vi "SonarBrake - Rev2.vi"() -> ()   [LabVIEW 2018]
uses:
  <vilib>/Platform/TimedLoop/XDataNode/timing_clust.ctl
  <vilib>/Platform/TimedLoop/XDataNode/nitl_modes.ctl
  <vilib>/Platform/TimedLoop/XDataNode/wakeup.ctl
  <vilib>/addons/control/pid/pid.llb/PID (DBL).vi
  <vilib>/platform/TimedLoop/XDataNode/XDataNode.xnode
  <vilib>/Platform/TimedLoop/XDataNode/XDNodeRunTimeDep.lvlib
  <vilib>/addons/control/pid/NI_PID_pid.lvlib
panel:
  in  "Reset":bool
  out "Diag":cluster{i32, i16, dbl, i16}(graph)={3, 0, 0.43266588939999995, 1}
  in  "Read Enable":T1={"Cal Status"=TRUE, "Orientation"=TRUE, "Gyro"=FALSE, "Accelerometer"=FALSE, "Quanterion"=FALSE, "Accel Mode"=enum."Linear", "Magnetometer"=FALSE, "Register Mode"=enum."Quaternion"}
  in  "Tab Control":enum32{"Sonar"}(tab)
  in  "Tol (sec)":dbl=0.25 format="%#_13g"
  in  "Tol (in)":dbl=1.1
  out "Arrived":bool
  out "Sonar Error":dbl=-4.3266588939999995
  in  "Rate Thresh":dbl=100.0 format="%#_13g"
  out "OOR":bool
  out "Mode":bool=TRUE
  in  "hi limit":dbl=200.0
  out "Strobe":bool
  in  "standoff":dbl=5.0 format="%.2f"
  out "Sonar Left":cluster{"Filtered":dbl, dbl}(graph)={"Filtered"=12.326658894, 12.326658894}
  out "Sonar Late?":bool
  out "Period":i64=40
  in  "Reset Enc":bool
  out "Enc":dbl=-31.431918913398693
  in  "Hyster":dbl=0.1 format="%#_13g"
  out "State":i32=3
  in  "reset IMU":bool
  in  "Test?":bool
  in  "clamp":cluster{"output high":dbl, "output low":dbl}={"output high"=1.0, "output low"=-1.0} {"output low" format="%.2f"; "output high" format="%.2f"}
  in  "Trans":dbl=14.0
  out "close":bool=TRUE
  in  "PID Sonar":T2={"proportional gain (Kc)"=0.035, "integral time (Ti, min)"=0.0, "derivative time (Td, min)"=0.001} {"derivative time (Td, min)" format="%.5f"; "integral time (Ti, min)" format="%.3f"; "proportional gain (Kc)" format="%.3f"}
  in  "Use Enc?":bool
  out "Sonar PID":cluster{"setpoint":dbl, "Filtered":dbl, i16}(graph)={"setpoint"=8.0, "Filtered"=12.326658894, 0}
  out "PID error":dbl=4.3266588939999995
  in  "scale enc":dbl=-0.04
  in  "db":dbl=0.04
  # "Real Time Data Repair"
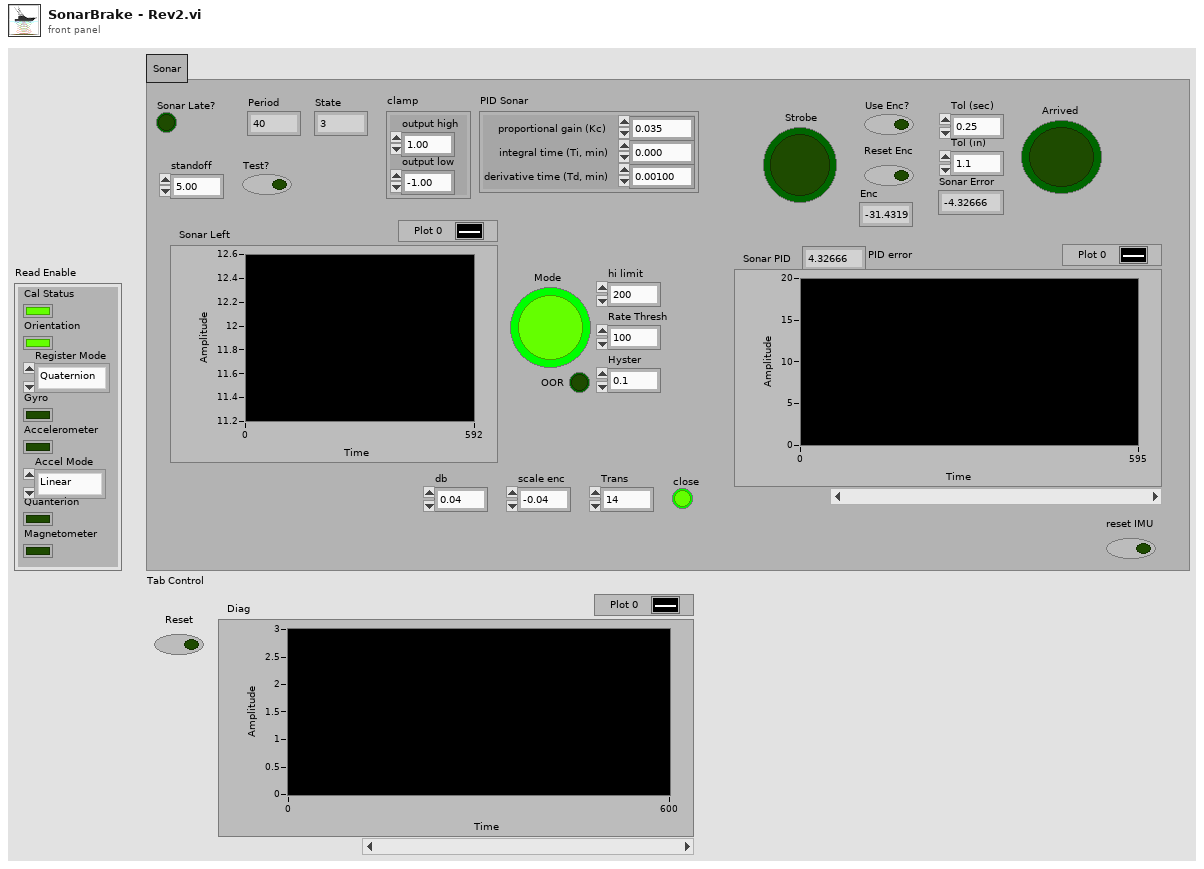
[diagram p1: front panel]
types:
  T1 = cluster{"Cal Status":bool, "Orientation":bool, "Gyro":bool, "Accelerometer":bool, "Quanterion":bool, "Accel Mode":enum8{"Raw Data", "Linear", "Gravity"}, "Magnetometer":bool, "Register Mode":enum8{"Euler", "Quaternion"}}
  T2 = cluster{"proportional gain (Kc)":dbl, "integral time (Ti, min)":dbl, "derivative time (Td, min)":dbl}
  T3 = typedef "ImuDevRef.ctl" = cluster{"I2CDevRef":T4, "Valid Cal File?":bool}
  T4 = typedef "WPI_I2CDevRef.ctl" = cluster{"DevStatus":errorcluster, "Device Address":u8, "Handle":i32, "I2C Bus":T5}
  T5 = typedef "i2c_bus.ctl" = enum16{"I2C On-Board", "I2C MXP", "Invalid"}
  T6 = typedef "XDNodeRunTimeDep.lvlib/timing_clust.ctl" = cluster{"Expected End [f-1]":u64, "Actual End [f-1]":u64, "Finished Late? [f-1]":bool, "Expected End [i-1]":u64, "Actual End [i-1]":u64, "Finished Late? [i-1]":bool, "Expected Start [i]":u64, "Actual Start [i]":u64, "Expected Start [f]":u64, "Actual Start [f]":u64, "Source Name":string, "Structure Name":string, "Period":i64, "Deadline":i64, "Offset":i64, "Start":i64, "Priority":i32, "Timeout":i32, "Mode":T7, "Wakeup Reason":T8, "Error":errorcluster, "Source Type":string, "Secondary Source Type":string, "Global End Time":u64, "Global Start Time":u64, "Frame Duration":u64, "Iteration Duration":u64, "Assigned CPU":i32, "I/O Scan Engine Mode":u32}
  T7 = typedef "XDNodeRunTimeDep.lvlib/nitl_modes.ctl" = enum32{"No Change", "Process missed periods, maintain original phase", "Discard missed periods, maintain original phase", "Process missed periods, ignore original phase", "Discard missed periods, ignore original phase"}
  T8 = typedef "XDNodeRunTimeDep.lvlib/wakeup.ctl" = enum32{"Normal", "Aborted", "Asynchronous wakeup", "Timing source error", "Timed loop error", "Timeout"}
  T9 = typedef "WPI_AnalogChannelDevRef.ctl" = cluster{"DevStatus":errorcluster, "Analog Channel":T10}
  T10 = typedef "FPGA_AIChannel.ctl" = enum8{"AI 0", "AI 1", "AI 2", "AI 3", "AI MXP 0", "AI MXP 1", "AI MXP 2", "AI MXP 3", "Invalid"}
  T11 = cluster{"Yaw":dbl, "Roll":dbl, "Pitch":dbl, "Yaw Wind":dbl, "Roll Wind":dbl, "Pitch Wind":dbl}
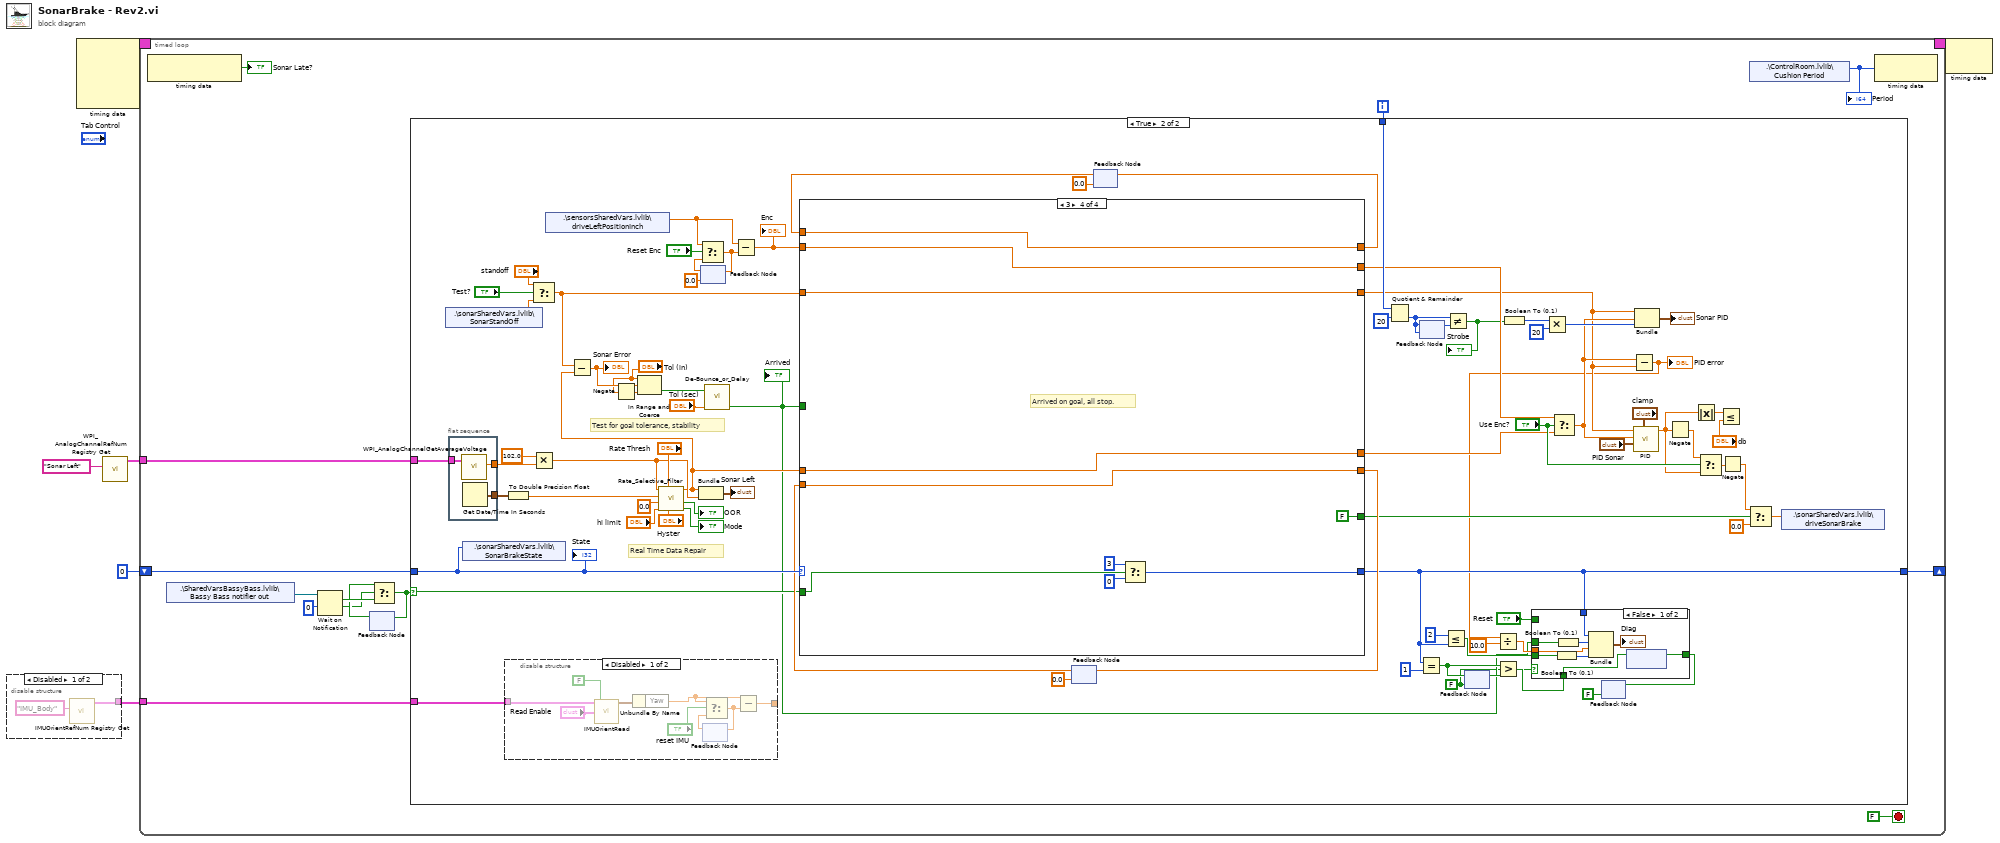
[diagram p0: block diagram]
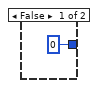
[diagram p3: hidden frame]
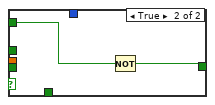
[diagram p4: hidden frame]
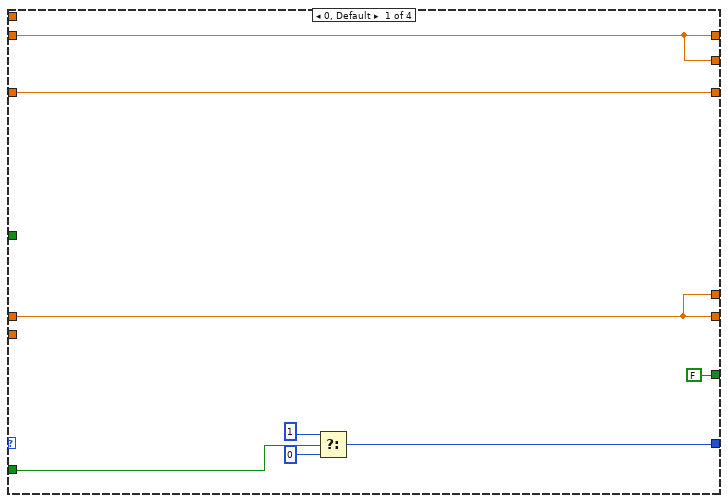
[diagram p6: hidden frame]
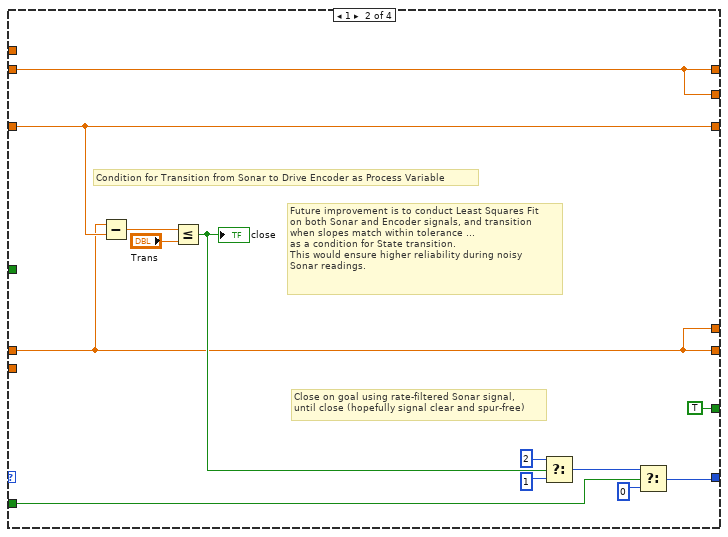
[diagram p7: hidden frame]
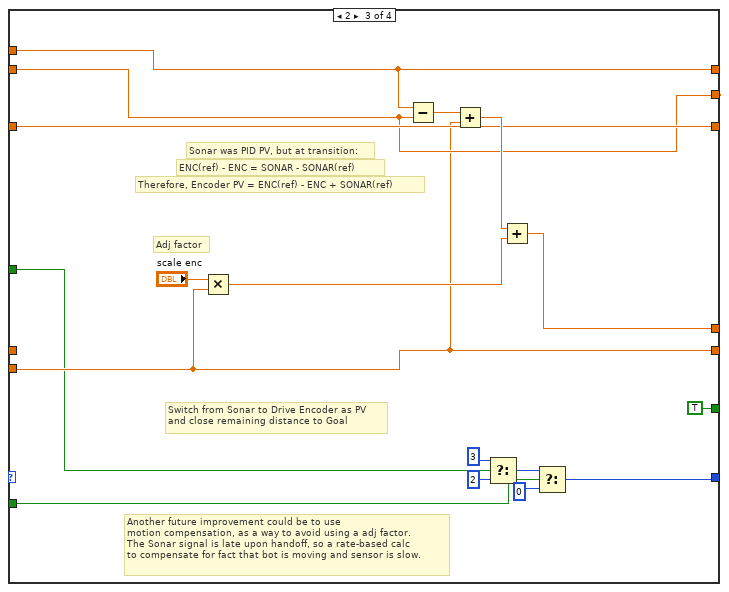
[diagram p8: hidden frame]
diagram:
  n1 = disable-structure shown="Disabled" {
    disable-tunnel: [w7 _] -> w1
    frame Disabled {
      n2 = call <userlib>:"IMUOrientRefNum Registry Get.vi"("refnum name"="IMU_Body") -> ("IMUDevRef out"=w7:T3)  [unwired: 9 in, 1 out]
    }
    frame Enabled {
    }
  }
  n3 = node-c288() -> (w6:T6)  [unwired: 4 in]
  n4 = call <vilib>:"WPI_AnalogChannelRefNum Registry Get.vi"("refnum name"="Sonar Left") -> ("AIDeviceRef"=w3:T9)  [unwired: 9 in, 1 out]
  n5 = timed-loop {
    timing: w6 -> [_]
    timing-out: [_] -> w5
    tunnel: w3 -> [w21]
    shift-right: [w15] -> _
    shift-left: 0 -> [w16]
    tunnel: w1 -> [w17]
    i -> [w19]
    stop <- FALSE stop-if-true
    n6 = node-c288() -> (→"Sonar Late?":bool)  [unwired: 1 in]
    n7 = shared-variable ".\\SharedVarsBassyBass.lvlib\\Bassy Bass notifier out"() -> (w14:refnum<notifier>)  [unwired: 1 in, 1 out]
    n8 = Wait on Notification(notifier=w14, timeout in ms (-1)=0) -> (notification=w12:bool, timed out?=w10:bool)  [unwired: 2 in, 2 out]
    n9 = feedback #1() -> (w11:bool)  [unwired: 1 in]
    n10 = Select(t=w11, s=w10, f=w12) -> (s? t:f=w9:bool)
    n11 = feedback-in #1(w9) -> ()
    n12 = case shown="True" w9 {
      selector: w9 -> [_ w30]
      tunnel: w21 -> [_ w101]
      tunnel: w19 -> [_ w97]
      tunnel: w17 -> [_ w74]
      tunnel: w16 -> [_ w68]
      tunnel: [0 ("t") w36] -> w15
      frame False {
      }
      frame True {
        w24 = FALSE ("Shock")
        # "Real Time Data Repair"
        # "Test for goal tolerance, stability"
        n13 = shared-variable ".\\sonarSharedVars.lvlib\\SonarStandOff"() -> (w71:dbl)  [unwired: 1 in, 1 out]
        n14 = flat-sequence {
          tunnel: [w124] -> w87
          tunnel: w101 -> [w123]
          tunnel: [w122] -> w94
          frame #0 {
            n15 = call <vilib>:"WPI_AnalogChannelGetAverageVoltage.vi"("AIDeviceRef"=w123) -> ("Voltage"=w124:dbl)  [unwired: 8 in, 2 out]
            n16 = Get Date/Time In Seconds() -> (seconds since 1Jan1904=w122:timestamp)
          }
        }
        n17 = shared-variable ".\\sonarSharedVars.lvlib\\SonarBrakeState"(w68) -> ()  [unwired: 1 in, 1 out]
        n18 = disable-structure shown="Disabled" {
          disable-tunnel: w74 -> [w114 _]
          disable-tunnel: [w113 _] -> _
          frame Disabled {
            n19 = call <userlib>:"IMUOrientRead.vi"("IMU Dev Ref"=w114, "Orient Reset (Wind)"=FALSE, "Read Enable"="Read Enable") -> ("Orient Y/R/P"=w119:T11)  [unwired: 5 in, 7 out]
            n20 = Unbundle By Name(w119) -> ("Yaw"=w115:dbl)
            n21 = feedback #2() -> (w118:dbl)  [unwired: 1 in]
            n22 = Select(t=w115, s="reset IMU", f=w118) -> (s? t:f=w117:dbl)
            n23 = feedback-in #2(w117) -> ()
            n24 = Subtract(x=w115, y=w117) -> (x-y=w113:dbl)
          }
          frame Enabled {
          }
        }
        n25 = To Double Precision Float(number=w94) -> (double precision float=w93:dbl)
        n26 = Select(t="standoff", s="Test?", f=w71) -> (s? t:f=w72:dbl)
        n27 = Multiply(x=102.0, y=w87) -> (x*y=w82:dbl)
        n28 = shared-variable ".\\sensorsSharedVars.lvlib\\driveLeftPositionInch"() -> (w75:dbl)  [unwired: 1 in, 1 out]
        n29 = Negate(x="Tol (in)") -> (-x=w85:dbl)
        n30 = call <userlib>:"Rate_Selective_Filter.vi"("Hyster"="Hyster", "Rate Thresh"="Rate Thresh", "hi limit"="hi limit", "lo limit"=0.0, "Time"=w93, "Distance"=w82) -> ("Mode"=→"Mode":bool, "OOR"=→"OOR":bool, "Filtered"=w76:dbl)  [unwired: 1 in]
        n31 = Subtract(x=w72, y=w76) -> (x-y=w86:dbl)
        "Sonar Error" <- w86
        n32 = In Range and Coerce(upper limit="Tol (in)", x=w86, lower limit=w85) -> (In Range?=w25:bool)  [unwired: 1 out]
        n33 = Bundle("Filtered"=w76, w82) -> (→"Sonar Left":cluster{"Filtered":dbl, dbl})  [unwired: 1 in]
        n34 = feedback #3(0.0) -> (w79:dbl)
        n35 = Select(t=w75, s="Reset Enc", f=w79) -> (s? t:f=w77:dbl)
        n36 = feedback-in #3(w77) -> ()
        n37 = call <userlib>:"De-Bounce_or_Delay.vi"("Eval Period (sec)"="Tol (sec)", "Signal Input"=w25) -> ("Stable"=w26:bool)  [unwired: 9 in]
        "Arrived" <- w26
        n38 = Subtract(x=w75, y=w77) -> (x-y=w78:dbl)
        "Enc" <- w78
        n39 = feedback #4(0.0 ("Filtered")) -> (w54:dbl)
        n40 = feedback #5(0.0) -> (w57:dbl)
        n41 = case shown="3" w68 {
          tunnel: [w131 w145 w161 w164] -> w36
          tunnel: w30 -> [w129 w144 w160 w163]
          tunnel: w72 -> [w128 w137 w151 w169]
          tunnel: w78 -> [w126 w134 w150 w170]
          tunnel: w76 -> [w125 w133 _ w168]
          tunnel: w26 -> [_ _ w147 _]
          tunnel: [w126 w134 w152 w171] -> w59
          tunnel: [w128 w137 w151 w169] -> w34
          tunnel: [w125 w133 w148 w167] -> w56
          tunnel: [w125 w133 w149 w168] -> w52
          tunnel: [w126 w134 w150 w170] -> w53
          tunnel: w57 -> [_ _ w152 w171]
          tunnel: w54 -> [_ _ w148 w167]
          tunnel: [FALSE TRUE TRUE FALSE] -> w48
          frame 0, Default {
            n42 = Select(t=1, s=w129, f=0) -> (s? t:f=w131:i32)
          }
          frame 1 {
            # "Close on goal using rate-filtered Sonar signal,\nuntil close (hopefully signal clear and spur-free)"
            # "Future improvement is to conduct Least Squares Fit\non both Sonar and Encoder signals, and transition\nwhen slopes match within tolerance ...\nas a condition for State transition.\nThis would ensure higher reliability during noisy\nSonar readings."
            # "Condition for Transition from Sonar to Drive Encoder as Process Variable"
            n43 = Subtract(x=w133, y=w137) -> (x-y=w138:dbl)
            n44 = Less Or Equal?(x=w138, y="Trans") -> (x <= y?=w136:bool)
            "close" <- w136
            n45 = Select(t=2, s=w136, f=1) -> (s? t:f=w140:i32)
            n46 = Select(t=w140, s=w144, f=0) -> (s? t:f=w145:i32)
          }
          frame 2 {
            # "Adj factor"
            # "Another future improvement could be to use \nmotion compensation, as a way to avoid using a adj factor.\nThe Sonar signal is late upon handoff, so a rate-based calc\nto compensate for fact that bot is moving and sensor is slow."
            # "Switch from Sonar to Drive Encoder as PV\nand close remaining distance to Goal"
            # "Sonar was PID PV, but at transition:"
            # "Therefore, Encoder PV = ENC(ref) - ENC + SONAR(ref)"
            # "ENC(ref) - ENC = SONAR - SONAR(ref)"
            n47 = Multiply(x="scale enc", y=w148) -> (x*y=w156:dbl)
            n48 = Subtract(x=w152, y=w150) -> (x-y=w159:dbl)
            n49 = Add(x=w159, y=w148) -> (x+y=w157:dbl)
            n50 = Select(t=3, s=w147, f=2) -> (s? t:f=w153:i32)
            n51 = Add(x=w157, y=w156) -> (x+y=w149:dbl)
            n52 = Select(t=w153, s=w160, f=0) -> (s? t:f=w161:i32)
          }
          frame 3 {
            # "Arrived on goal, all stop."
            n53 = Select(t=3, s=w163, f=0) -> (s? t:f=w164:i32)
          }
        }
        n54 = feedback-in #4(w56) -> ()
        n55 = feedback-in #5(w59) -> ()
        n56 = Quotient & Remainder(x=w97, y=20) -> (floor(x/y)=w100:i32)  [unwired: 1 out]
        n57 = Equal?(x=w36, y=1) -> (x = y?=w41:bool)
        n58 = feedback #6(w100) -> (w99:i32)
        n59 = feedback-in #6(w100) -> ()
        n60 = Less Or Equal?(x=2, y=w36) -> (x <= y?=w37:bool)
        n61 = Not Equal?(x=w100, y=w99) -> (x != y?=w47:bool)
        "Strobe" <- w47
        n62 = feedback #7(w24) -> (w43:bool)
        n63 = feedback-in #7(w41) -> ()
        n64 = Greater?(x=w41, y=w43) -> (0:w42:bool)
        n65 = Boolean To (0,1)(Boolean=w47) -> (0, 1=w66:i16)
        n66 = Multiply(x=w66, y=i16 20) -> (x*y=w62:i16)
        n67 = Select(t=w53, s="Use Enc?", f=w52) -> (s? t:f=w35:dbl)
        n68 = feedback #8(FALSE) -> ()  [unwired: 1 in]
        n69 = Subtract(x=w35, y=w34) -> (x-y=w33:dbl)
        "PID error" <- w33
        n70 = Divide(x=w33, y=10.0) -> (x/y=w39:dbl)
        n71 = case shown="False" w24 {
          tunnel: w36 -> [w109 _]
          tunnel: w26 -> [w107 _]
          tunnel: w39 -> [w106 _]
          tunnel: "Reset" -> [_ w112]
          tunnel: [w105 w111] -> w32
          tunnel: w42 -> [w104 _]
          tunnel: w37 -> [w102 _]
          frame False {
            n72 = Boolean To (0,1)(Boolean=w102) -> (0, 1=w103:i16)
            n73 = Boolean To (0,1)(Boolean=w107) -> (0, 1=w108:i16)
            n74 = Bundle("t"=w109, w108, w106, w103) -> (→"Diag":cluster{"t":i32, i16, dbl, i16})  [unwired: 1 in]
            n75 = feedback #9() -> (w105:bool)  [unwired: 1 in]
            n76 = feedback-in #9(w104) -> ()
          }
          frame True {
            n77 = Not(x=w112) -> (.not. x?=w111:bool)
          }
        }
        n78 = feedback-in #8(w32) -> ()
        n79 = call-poly <vilib>:"PID.vi"("output range"="clamp", "PID gains"="PID Sonar", "process variable"=w35, "setpoint"=w34) -> ("output"=w29:dbl)  [unwired: 6 in, 1 out]
        n80 = Bundle("Double"=w34, "Filtered"=w35, w62) -> (→"Sonar PID":cluster{"Double":dbl, "Filtered":dbl, i16})  [unwired: 1 in]
        n81 = Negate(x=w29) -> (-x=w61:dbl)
        n82 = Absolute Value(x=w29) -> (abs(x)=w28:dbl)
        n83 = Select(t=w61, s="Use Enc?", f=w29) -> (s? t:f=w31:dbl)
        n84 = Less Or Equal?(x=w28, y="db") -> ()  [unwired: 1 out]
        n85 = Negate(x=w31) -> (-x=w51:dbl)
        n86 = Select(t=w51, s=w48, f=0.0) -> (s? t:f=w50:dbl)
        n87 = shared-variable ".\\sonarSharedVars.lvlib\\driveSonarBrake"(w50) -> ()  [unwired: 1 in, 1 out]
        "State" <- w68
      }
    }
    n88 = shared-variable ".\\ControlRoom.lvlib\\Cushion Period"() -> (w18:i64)  [unwired: 1 in, 1 out]
    "Period" <- w18
    n89 = node-c288(w18) -> ()  [unwired: 1 out]
  }
  n90 = node-c288(w5) -> ()  [unwired: 1 out]
